vi "WindSpeedToLabel.vi"(10 "Wind speed (m/sec)":sgl) -> (2 "Label":string="Calm")   [LabVIEW 2015]
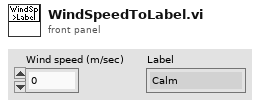
[diagram p1: front panel]
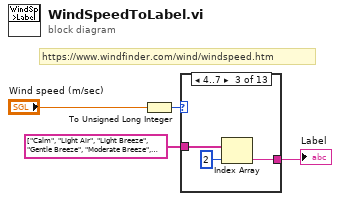
[diagram p0: block diagram]
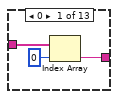
[diagram p2: hidden frame]
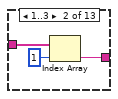
[diagram p3: hidden frame]
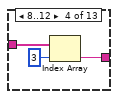
[diagram p4: hidden frame]
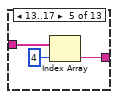
[diagram p5: hidden frame]
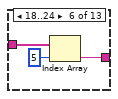
[diagram p6: hidden frame]
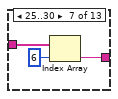
[diagram p7: hidden frame]
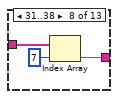
[diagram p8: hidden frame]
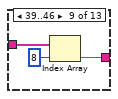
[diagram p9: hidden frame]
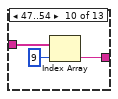
[diagram p10: hidden frame]
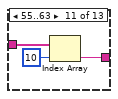
[diagram p11: hidden frame]
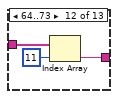
[diagram p12: hidden frame]
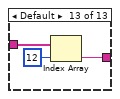
[diagram p13: hidden frame]
diagram:
  # "https://www.windfinder.com/wind/windspeed.htm"
  n1 = To Unsigned Long Integer(number="Wind speed (m/sec)") -> (unsigned 32bit integer=w2:u32)
  n2 = case shown="4..7" w2 {
    tunnel: string[] ["Calm", "Light Air", "Light Breeze", "Gentle Breeze", "Moderate Breeze", "Fresh Breeze", "Strong Breeze", "Near Gale", "Gale", "Severe Gale", "Storm", "Violent Storm", "Hurricane"] -> [w7 w10 w13 w16 w19 w22 w25 w28 w31 w34 w37 w40 w43]
    tunnel: [w5 w8 w11 w14 w17 w20 w23 w26 w29 w32 w35 w38 w41] -> w4
    frame 0 {
      n3 = Index Array(array=w7, index=0) -> (element=w5:string)
    }
    frame 1..3 {
      n4 = Index Array(array=w10, index=1) -> (element=w8:string)
    }
    frame 4..7 {
      n5 = Index Array(array=w13, index=2) -> (element=w11:string)
    }
    frame 8..12 {
      n6 = Index Array(array=w16, index=3) -> (element=w14:string)
    }
    frame 13..17 {
      n7 = Index Array(array=w19, index=4) -> (element=w17:string)
    }
    frame 18..24 {
      n8 = Index Array(array=w22, index=5) -> (element=w20:string)
    }
    frame 25..30 {
      n9 = Index Array(array=w25, index=6) -> (element=w23:string)
    }
    frame 31..38 {
      n10 = Index Array(array=w28, index=7) -> (element=w26:string)
    }
    frame 39..46 {
      n11 = Index Array(array=w31, index=8) -> (element=w29:string)
    }
    frame 47..54 {
      n12 = Index Array(array=w34, index=9) -> (element=w32:string)
    }
    frame 55..63 {
      n13 = Index Array(array=w37, index=10) -> (element=w35:string)
    }
    frame 64..73 {
      n14 = Index Array(array=w40, index=11) -> (element=w38:string)
    }
    frame Default {
      n15 = Index Array(array=w43, index=12) -> (element=w41:string)
    }
  }
  "Label" <- w4
